vi "Write Cells.vi"(8 "error in":errorcluster, 10 "Cells":refnum<class "PAS Cell.lvclass">[](array[class]), 11 "PAS in":refnum<class "PAS.lvclass">) -> (0 "error out":errorcluster, 3 "PAS out":refnum<class "PAS.lvclass">)   [LabVIEW 2015, in "PAS Library.lvlib" / "PAS.lvclass"]
uses:
  PAS.lvclass
  Cell/PAS Cell.lvclass
  PAS.lvclass/PAS.ctl
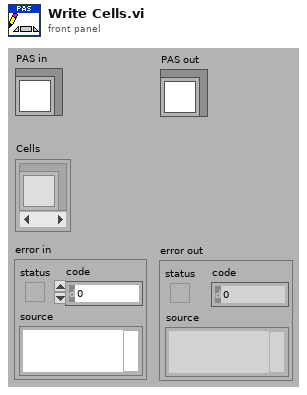
[diagram p1: front panel]
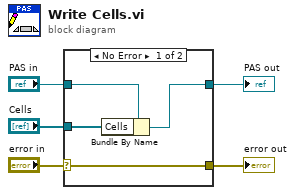
[diagram p0: block diagram]
diagram:
  n1 = case shown="No Error" "error in" {
    selector: "error in" -> [w9 w10]
    tunnel: [w9 w10] -> w4
    tunnel: [w7 w11] -> w2
    tunnel: "PAS in" -> [w8 w11]
    tunnel: "Cells" -> [w6 _]
    frame No Error {
      n2 = Bundle By Name(cluster=w8, "Cells"=w6) -> (w7:refnum<class "PAS.lvclass">)
    }
    frame Error {
    }
  }
  "error out" <- w4
  "PAS out" <- w2
